vi "Send Dashboard Data.vi"   [LabVIEW 2012]
uses:
  BotStatus.vi
types:
  T1 = typedef "WPI_EncoderDevRef.ctl" = cluster{"DevStatus":errorcluster, "EncoderIndex":T2, "CounterIndex":T3, "DistancePerCount":dbl, "Decoding Type":T4}
  T2 = typedef "FPGA_EncoderIdx.ctl" = enum8{"Enc 0", "Enc 1", "Enc 2", "Enc 3", "Invalid"}
  T3 = typedef "FPGA_CounterCtrSystemIndex.ctl" = enum8{"Ctr 0", "Ctr 1", "Ctr 2", "Ctr 3", "Ctr 4", "Ctr 5", "Ctr 6", "Ctr 7", "Invalid"}
  T4 = typedef "WPI_EncoderType.ctl" = enum16{"1x", "2x", "4x"}
  T5 = typedef "WPI_ServoDeviceRef.ctl" = cluster{"DeviceStatus":errorcluster, "Digital Module":T6, "PWM Channel":T7, "DeadBand":T8}
  T6 = typedef "FPGA_TypedefDigitalModule.ctl" = enum16{"Digital Module 1", "Digital Module 2"}
  T7 = typedef "FPGA_DIOPWMChannel.ctl" = enum8{"PWM 1", "PWM 2", "PWM 3", "PWM 4", "PWM 5", "PWM 6", "PWM 7", "PWM 8", "PWM 9", "PWM 10", "Invalid"}
  T8 = typedef "WPI_PWMDeadband.ctl" = cluster{"Name":string, "maxPositivePwm":i32, "minPositivePwm":i32, "centerPwm":i32, "maxNegativePwm":i32, "minNegativePwm":i32, "angularRange":u16}
  T9 = cluster{"Middle":bool, "InCannon":bool, "InFlipper":bool, "Bottom":bool, "FlipperDown":bool}
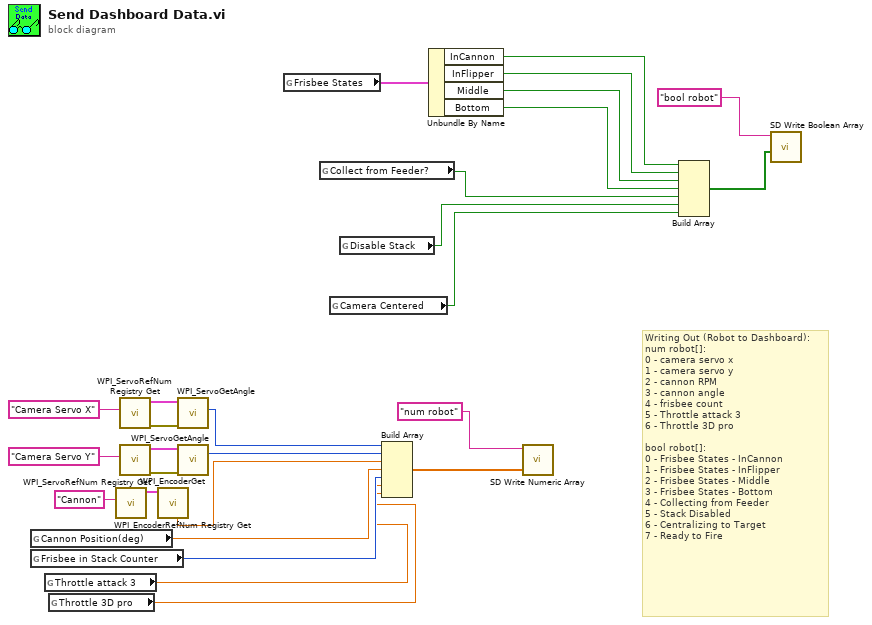
[diagram p0: block diagram]
diagram:
  # "Writing Out (Robot to Dashboard):\nnum robot[]:\n0 - camera servo x\n1 - camera servo y\n2 - cannon RPM\n3 - cannon angle\n4 - frisbee count\n5 - Throttle attack 3\n6 - Throttle 3D pro\n\nbool robot[]:\n0 - Frisbee States - InCannon\n1 - Frisbee States - InFlipper\n2 - Frisbee States - Middle\n3 - Frisbee States - Bottom\n4 - Collecting from Feeder\n5 - Stack Disabled\n6 - Centralizing to Target\n7 - Ready to Fire"
  n1 = global read "BotStatus.vi" "Cannon Position(deg)"() -> (w13:dbl)
  n2 = global read "BotStatus.vi" "Frisbee in Stack Counter"() -> (w14:i32)
  n3 = global read "BotStatus.vi" "Throttle attack 3"() -> (w2:dbl)
  n4 = global read "BotStatus.vi" "Throttle 3D pro"() -> (w1:dbl)
  n5 = call <vilib>:"WPI_EncoderRefNum Registry Get.vi"("refnum name"="Cannon") -> ("EncoderDevRef"=w17:T1)  [unwired: 9 in, 1 out]
  n6 = call <vilib>:"WPI_ServoRefNum Registry Get.vi"("refnum name"="Camera Servo X") -> ("error out"=w24:errorcluster, "ServoDeviceRef"=w25:T5)  [unwired: 9 in]
  n7 = call <vilib>:"WPI_ServoRefNum Registry Get.vi"("refnum name"="Camera Servo Y") -> ("error out"=w20:errorcluster, "ServoDeviceRef"=w21:T5)  [unwired: 9 in]
  n8 = call <vilib>:"WPI_EncoderGet.vi"("EncoderDevRef"=w17) -> ("Rate"=w15:dbl)  [unwired: 5 in, 5 out]
  n9 = call <vilib>:"WPI_ServoGetAngle.vi"("ServoDeviceRef"=w25, "error in (no error)"=w24) -> ("Angle"=w19:u16)  [unwired: 6 in, 2 out]
  n10 = call <vilib>:"WPI_ServoGetAngle.vi"("ServoDeviceRef"=w21, "error in (no error)"=w20) -> ("Angle"=w18:u16)  [unwired: 6 in, 2 out]
  n11 = global read "BotStatus.vi" "Frisbee States"() -> (w27:T9)
  n12 = global read "BotStatus.vi" "Collect from Feeder?"() -> (w6:bool)
  n13 = global read "BotStatus.vi" "Camera Centered"() -> (w4:bool)
  n14 = global read "BotStatus.vi" "Disable Stack"() -> (w5:bool)
  n15 = Build Array(w19, w18, w15, w13, w14, w2, w1) -> (w12:dbl[])
  n16 = Unbundle By Name(w27) -> ("InCannon"=w10:bool, "InFlipper"=w9:bool, "Middle"=w8:bool, "Bottom"=w7:bool)
  n17 = call <vilib>:"SD Write Numeric Array.vi"("Numeric Array"=w12, "Name"="num robot") -> ()  [unwired: 8 in, 2 out]
  n18 = Build Array(w10, w9, w8, w7, w6, w5, w4) -> (w3:bool[])
  n19 = call <vilib>:"SD Write Boolean Array.vi"("Boolean Array"=w3, "Name"="bool robot") -> ()  [unwired: 8 in, 2 out]
